vi "Enter Field (No Objects).vi"(7 "Field monitor":refnum<vi>, 8 "error in (no error)":errorcluster, 10 "Target field":dbl[unit], 11 "Cluster In":T4={"Field"=0.0, "Rate"=0.0, "Status"={"Sweeping"=FALSE, "Clamped"=FALSE, "Hold"=FALSE, "At Rest"=FALSE, "Quench"=FALSE, "Persistent Mode"=FALSE, "Switch Heater"=FALSE}, "ILM Shut Down?"=FALSE, "IO Info"={"Address"={"Com Port"=1, "ISOBUS Address"=2, "GPIB Address"=24, "Communication"=enum."ISOBUS"}, "Version"=enum."IPS"}, "IO Info (Level Meter)"={"Address"={"Com Port"=1, "ISOBUS Address"=5, "GPIB Address"=24, "Communication"=enum."ISOBUS"}, "ILM Name"="", "Display Channel"=[]}, "Training?"=FALSE, "Training Field and Speed Cluster"={"Training Field"=[0.0, 4.108, 5.78, 8.001], "Training Speed"=[0.0057, 0.0022833333333333334, 0.0011333333333333334, 0.0011333333333333334]}}) -> (0 "error out":errorcluster, 3 "Cluster Out":T4={"Field"=0.0, "Rate"=0.0, "Status"={"Sweeping"=FALSE, "Clamped"=FALSE, "Hold"=FALSE, "At Rest"=FALSE, "Quench"=FALSE, "Persistent Mode"=FALSE, "Switch Heater"=FALSE}, "ILM Shut Down?"=FALSE, "IO Info"={"Address"={"Com Port"=1, "ISOBUS Address"=2, "GPIB Address"=24, "Communication"=enum."ISOBUS"}, "Version"=enum."IPS"}, "IO Info (Level Meter)"={"Address"={"Com Port"=1, "ISOBUS Address"=5, "GPIB Address"=24, "Communication"=enum."ISOBUS"}, "ILM Name"="", "Display Channel"=[]}, "Training?"=FALSE, "Training Field and Speed Cluster"={"Training Field"=[0.0, 4.108, 5.78, 8.001], "Training Speed"=[0.0057, 0.0022833333333333334, 0.0011333333333333334, 0.0011333333333333334]}})   [LabVIEW 2009]
doc: "Establish an initial magnetic field - perhaps starting at zero or some other point. Use this SubVI for large (not incremental) field adjustments."
uses:
  Magnet status.ctl
  Oxford/PSSUBS.LLB/PSIO.ctl
  Oxford/BUSGEN.LLB/OxfordAddress.ctl
  Power Supply.lvclass
panel:
  in  "Dummy field monitor":dbl[unit]
  in  "Status display":refnum<vi>
  in  "resetrate?":bool
  out "canceled?":bool
  in  "cancel":bool
  out "disp":string
  out "fieldOUT":dbl[unit]
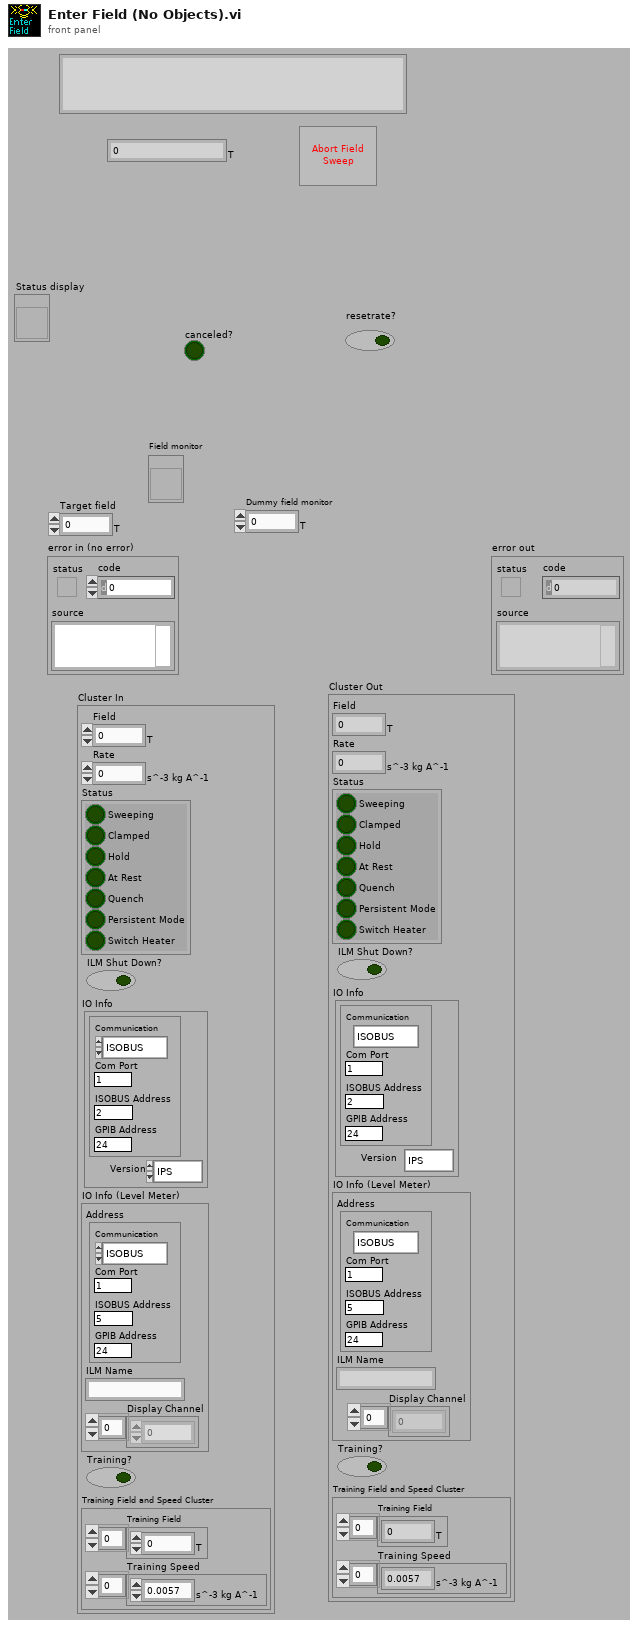
[diagram p1: front panel]
types:
  T1 = typedef "Power Supply.lvclass/Magnet status.ctl" = cluster{"Sweeping":bool, "Clamped":bool, "Hold":bool, "At Rest":bool, "Quench":bool, "Persistent Mode":bool, "Switch Heater":bool}
  T2 = typedef "PSIO.ctl" = cluster{"Address":T3, "Version":enum16{"PS", "IPS"}}
  T3 = typedef "OxfordAddress.ctl" = cluster{"Com Port":i32, "ISOBUS Address":i32, "GPIB Address":i16, "Communication":enum16{"RS232", "ISOBUS", "GPIB", "Gateway"}}
  T4 = cluster{"Field":dbl[unit], "Rate":dbl[unit], "Status":T1, "ILM Shut Down?":bool, "IO Info":T2, "IO Info (Level Meter)":cluster{"Address":T3, "ILM Name":string, "Display Channel":i32[]}, "Training?":bool, "Training Field and Speed Cluster":cluster{"Training Field":dbl[unit][], "Training Speed":dbl[unit][]}}
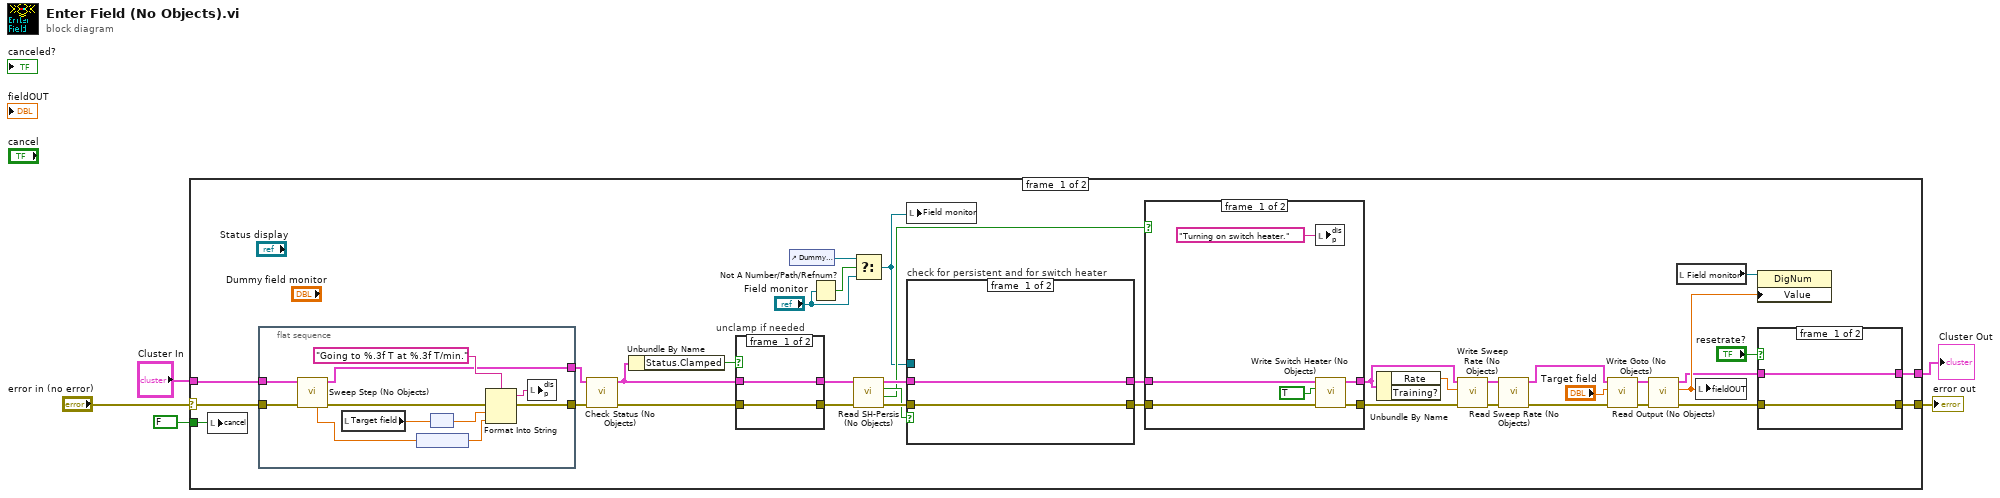
[diagram p0: block diagram]
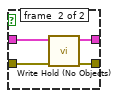
[diagram p3: hidden frame]
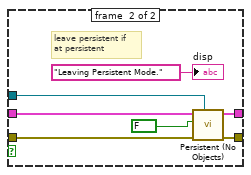
[diagram p4: hidden frame]
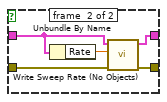
[diagram p5: hidden frame]
diagram:
  n1 = case shown="No Error" "error in (no error)" {
    selector: "error in (no error)" -> [w18 w85]
    tunnel: [w42 w85] -> w3
    tunnel: [w41 w84] -> w1
    tunnel: "Cluster In" -> [w16 w84]
    tunnel: FALSE ("cancel") -> [w24 _]
    frame #0 {
      n2 = local write "cancel"(w24) -> ()
      n3 = flat-sequence {
        tunnel: w18 -> [w50]
        tunnel: [w51] -> w17
        tunnel: w16 -> [w43]
        tunnel: [w48] -> w11
        frame #0 {
          n4 = call "Sweep Step (No Objects).vi"("error in (no error)"=w50, "Cluster In"=w43) -> ("error out"=w49:errorcluster, "Cluster Out"=w48:T4, "rate"=w45:dbl[unit])  [unwired: 5 in, 2 out]
          n5 = local read "Target field"() -> (w47:dbl[unit])
          n6 = node(w45) -> (w44:dbl)
          n7 = node(w47) -> (w46:dbl)
          n8 = Format Into String(format string="Going to %.3f T at %.3f T/min.", error in=w49, w46, w44) -> (resulting string=w53:string, error out=w51:errorcluster)  [unwired: 1 in]
          n9 = local write "disp"(w53) -> ()
        }
      }
      n10 = call "Check Status (No Objects).vi"("error in (no error)"=w17, "Cluster In"=w11) -> ("error out"=w30:errorcluster, "Cluster Out"=w31:T4)  [unwired: 6 in, 2 out]
      n11 = Unbundle By Name(w31) -> ("Status.Clamped"=w32:bool)
      n12 = case "unclamp if needed" shown="True" w32 {
        tunnel: w31 -> [w63 w64]
        tunnel: [w63 w67] -> w10
        tunnel: w30 -> [w62 w66]
        tunnel: [w62 w65] -> w36
        frame #0 {
        }
        frame #1 {
          n13 = call "Write Hold (No Objects).vi"("error in (no error)"=w66, "Cluster In"=w64) -> ("error out"=w65:errorcluster, "Cluster Out"=w67:T4)  [unwired: 8 in]
        }
      }
      n14 = control-ref of="Dummy field monitor"() -> (w21:refnum<vi>)
      n15 = Not A Number/Path/Refnum?(number/path/refnum="Field monitor") -> (NaN/Path/Refnum?=w23:bool)
      n16 = Select(t=w21, s=w23, f="Field monitor") -> (s? t:f=w20:refnum<vi>)
      n17 = call "Read SH-Persis (No Objects).vi"("error in (no error)"=w36, "Cluster In"=w10) -> ("error out"=w34:errorcluster, "SHon?"=w25:bool, "pers?"=w33:bool, "Cluster Out"=w35:T4)  [unwired: 4 in, 2 out]
      n18 = local write "Field monitor"(w20) -> ()
      n19 = case "check for persistent and for switch heater" shown="True" w33 {
        tunnel: w35 -> [w69 w70]
        tunnel: [w69 w73] -> w28
        tunnel: w34 -> [w68 w75]
        tunnel: [w68 w74] -> w27
        tunnel: w20 -> [_ w71]
        frame #0 {
        }
        frame #1 {
          # "leave persistent if\nat persistent"
          n20 = call "Persistent (No Objects).vi"("Field monitor ref"=w71, "error in (no error)"=w75, "Go to persistent mode?"=FALSE, "Cluster In"=w70) -> ("error out"=w74:errorcluster, "Cluster Out"=w73:T4)  [unwired: 6 in]
          "disp" <- "Leaving Persistent Mode."
        }
      }
      n21 = case shown="False" w25 {
        tunnel: w28 -> [w54 w60]
        tunnel: [w59 w60] -> w9
        tunnel: w27 -> [w58 w61]
        tunnel: [w57 w61] -> w26
        frame #0 {
          n22 = local write "disp"("Turning on switch heater." ("disp")) -> ()
          n23 = call "Write Switch Heater (No Objects).vi"("error in (no error)"=w58, "Turn SH On?"=TRUE, "Cluster In"=w54) -> ("error out"=w57:errorcluster, "Cluster Out"=w59:T4)  [unwired: 7 in]
        }
        frame #1 {
        }
      }
      n24 = Unbundle By Name(w9) -> ("Rate"=w29:dbl[unit])  [unwired: 1 out]
      n25 = call "Write Sweep Rate (No Objects).vi"("error in (no error)"=w26, "rate"=w29, "Cluster In"=w9) -> ("error out"=w38:errorcluster, "Cluster Out"=w8:T4)  [unwired: 7 in]
      n26 = call "Read Sweep Rate (No Objects).vi"("error in (no error)"=w38, "Cluster In"=w8) -> ("error out"=w37:errorcluster, "Cluster Out"=w7:T4)  [unwired: 7 in, 1 out]
      n27 = call "Write Goto (No Objects).vi"("error in (no error)"=w37, "Target"="Target field", "Cluster In"=w7) -> ("error out"=w12:errorcluster, "Cluster Out"=w6:T4)  [unwired: 7 in]
      n28 = call "Read Output (No Objects).vi"("error in (no error)"=w12, "Cluster In"=w6) -> ("error out"=w13:errorcluster, "Field"=w15:dbl[unit], "Cluster Out"=w14:T4)  [unwired: 6 in, 1 out]
      n29 = local read "Field monitor"() -> (w39:refnum<vi>)
      n30 = local write "fieldOUT"(w15) -> ()
      n31 = property class="DigNum"(reference=w39, "Value"=w15) -> ()  [unwired: 1 in, 2 out]
      n32 = case shown="True" "resetrate?" {
        tunnel: w14 -> [w78 w79]
        tunnel: w13 -> [w77 w83]
        tunnel: [w77 w82] -> w42
        tunnel: [w78 w81] -> w41
        frame #0 {
        }
        frame #1 {
          n33 = Unbundle By Name(w79) -> ("Rate"=w80:dbl[unit])
          n34 = call "Write Sweep Rate (No Objects).vi"("error in (no error)"=w83, "rate"=w80, "Cluster In"=w79) -> ("error out"=w82:errorcluster, "Cluster Out"=w81:T4)  [unwired: 7 in]
        }
      }
    }
    frame #1 {
    }
  }
  "error out" <- w3
  "Cluster Out" <- w1
